vi "Report data in.vi"() -> (2 "Report data":string[](array[string]))   [LabVIEW 2015]
uses:
  Galobal variable_TI.vi
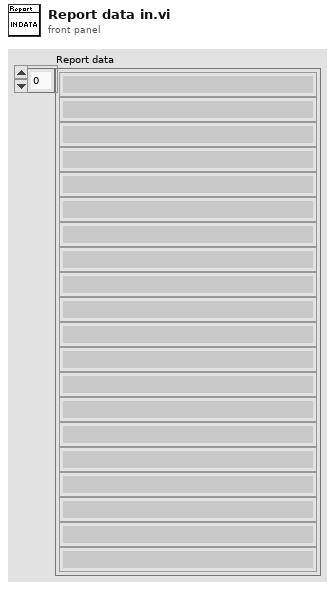
[diagram p1: front panel]
types:
  T1 = cluster{"IL Sensor1_Max AI0":dbl, "IL Sensor1_Min AI0":dbl, "IL Sensor1_Max AI1":dbl, "IL Sensor1_ Min AI1":dbl, "IL Sensor_Max (AI9)":dbl, "IL Sensor_Min  (AI9)":dbl, "IL Sensor_Max (AI10)":dbl, "IL Sensor_Min(AI10)":dbl, "IL Sensor_Max (AI11)":dbl, "IL Sensor_Min (AI11)":dbl, "IL Sensor_Max (AI12)":dbl, "IL Sensor_Min (AI12":dbl}
  T2 = cluster{"IL Sensor1_AI0":dbl, "IL Sensor1_AI1":dbl, "IL Sensor (AI6)":dbl, "IL Sensor  (AI7)":dbl, "IL Sensor (AI8)":dbl, "IL Sensor  (AI9)":dbl, "IL Sensor1_AI0":bool, "IL Sensor1_AI1":bool, "IL Sensor1_AI9":bool, "IL Sensor1_AI10":bool, "IL Sensor1_AI11":bool, "IL Sensor1_AI12":bool}
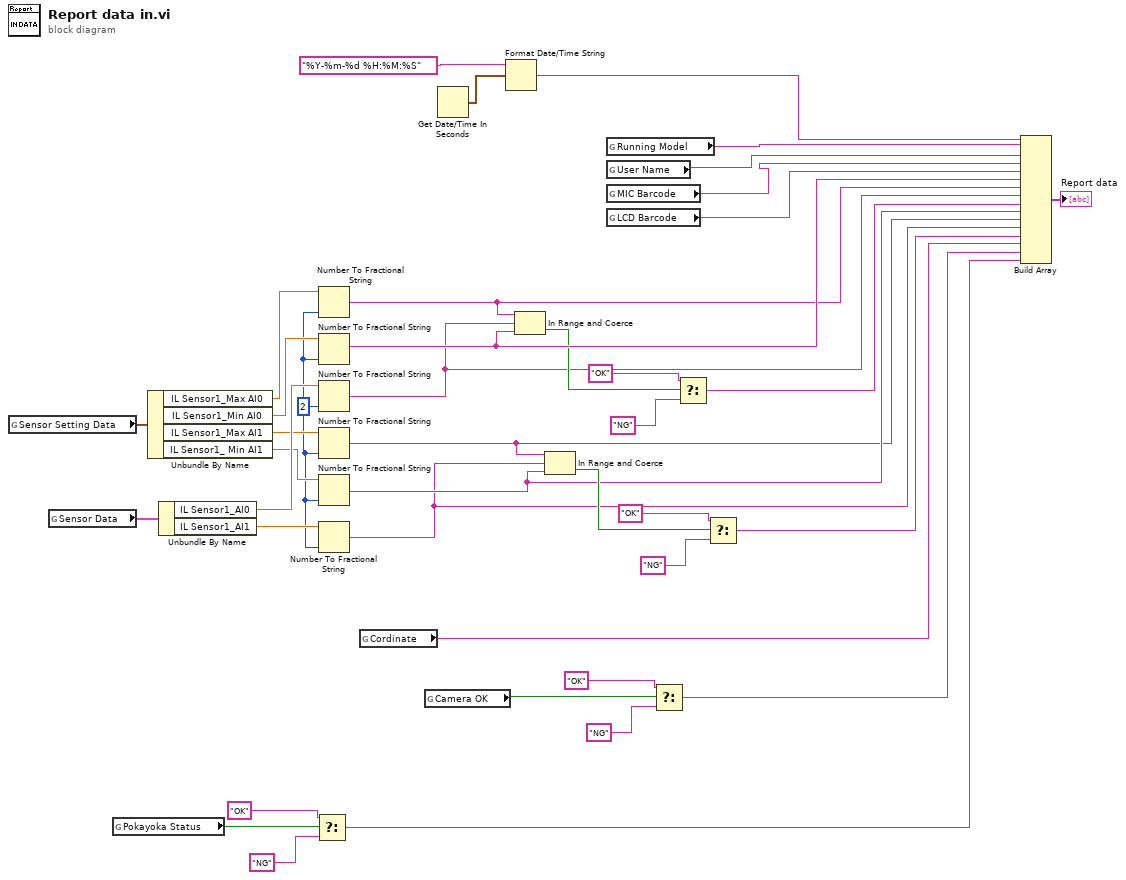
[diagram p0: block diagram]
diagram:
  w20 = i16 2 ("precision (6)")
  n1 = global read "Galobal variable_TI.vi" "Sensor Setting Data"() -> (w34:T1)
  n2 = global read "Galobal variable_TI.vi" "Sensor Data"() -> (w39:T2)
  n3 = global read "Galobal variable_TI.vi" "Pokayoka Status"() -> (w30:bool)
  n4 = Unbundle By Name(w34) -> ("IL Sensor1_Max AI0"=w35:dbl, "IL Sensor1_Min AI0"=w36:dbl, "IL Sensor1_Max AI1"=w37:dbl, "IL Sensor1_ Min AI1"=w38:dbl)
  n5 = Unbundle By Name(w39) -> ("IL Sensor1_AI0"=w40:dbl, "IL Sensor1_AI1"=w31:dbl)
  n6 = Select(t="OK" ("Camera Co-ordinate Max Value"), s=w30, f="NG" ("Camera Co-ordinate Max Value")) -> (s? t:f=w2:string)
  n7 = Number To Fractional String(number=w35, precision (6)=w20) -> (F-format string=w21:string)  [unwired: 2 in]
  n8 = Number To Fractional String(number=w36, precision (6)=w20) -> (F-format string=w22:string)  [unwired: 2 in]
  n9 = Number To Fractional String(number=w40, precision (6)=w20) -> (F-format string=w13:string)  [unwired: 2 in]
  n10 = Number To Fractional String(number=w37, precision (6)=w20) -> (F-format string=w10:string)  [unwired: 2 in]
  n11 = Number To Fractional String(number=w38, precision (6)=w20) -> (F-format string=w11:string)  [unwired: 2 in]
  n12 = Number To Fractional String(number=w31, precision (6)=w20) -> (F-format string=w9:string)  [unwired: 2 in]
  n13 = global read "Galobal variable_TI.vi" "Cordinate"() -> (w7:string)
  n14 = global read "Galobal variable_TI.vi" "Camera OK"() -> (w4:bool)
  n15 = Get Date/Time In Seconds() -> (seconds since 1Jan1904=w33:timestamp)
  n16 = Format Date/Time String(time format string (%c)="%Y-%m-%d %H:%M:%S", seconds (now)=w33) -> (date/time string=w27:string)  [unwired: 1 in]
  n17 = In Range and Coerce(upper limit=w21, x=w13, lower limit=w22) -> (In Range?=w17:bool)  [unwired: 1 out]
  n18 = In Range and Coerce(upper limit=w10, x=w9, lower limit=w11) -> (In Range?=w16:bool)  [unwired: 1 out]
  n19 = global read "Galobal variable_TI.vi" "Running Model"() -> (w26:string)
  n20 = global read "Galobal variable_TI.vi" "User Name"() -> (w25:string)
  n21 = global read "Galobal variable_TI.vi" "MIC Barcode"() -> (w24:string)
  n22 = global read "Galobal variable_TI.vi" "LCD Barcode"() -> (w23:string)
  n23 = Select(t="OK" ("Camera Co-ordinate Max Value"), s=w4, f="NG" ("Camera Co-ordinate Max Value")) -> (s? t:f=w3:string)
  n24 = Select(t="OK" ("Camera Co-ordinate Max Value"), s=w17, f="NG" ("Camera Co-ordinate Max Value")) -> (s? t:f=w12:string)
  n25 = Select(t="OK" ("Camera Co-ordinate Max Value"), s=w16, f="NG" ("Camera Co-ordinate Max Value")) -> (s? t:f=w8:string)
  n26 = Build Array(w27, w26, w25, w24, w23, w22, w21, w13, w12, w11, w10, w9, w8, w7, w3, w2) -> (→"Report data":string[])
